vi "Test_FGV1.vi"() -> (0 "output":dbl)   [LabVIEW 2017]
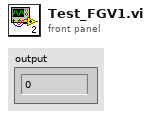
[diagram p1: front panel]
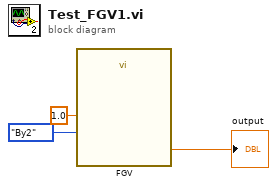
[diagram p0: block diagram]
diagram:
  n1 = call "FGV.vi"("input"=1.0, "mode"=enum16{"By1", "By2"}."By2") -> ("output"=→"output":dbl)  [unwired: 9 in]
